vi "Detele_repeated.vi"(11 "timetags":u32[][](array[numeric])) -> (3 "detections":cluster{"time_ns":u32[], "q_photons":u32[]})   [LabVIEW 2014]
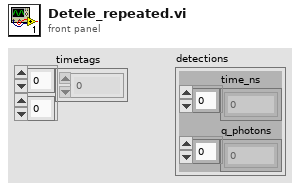
[diagram p1: front panel]
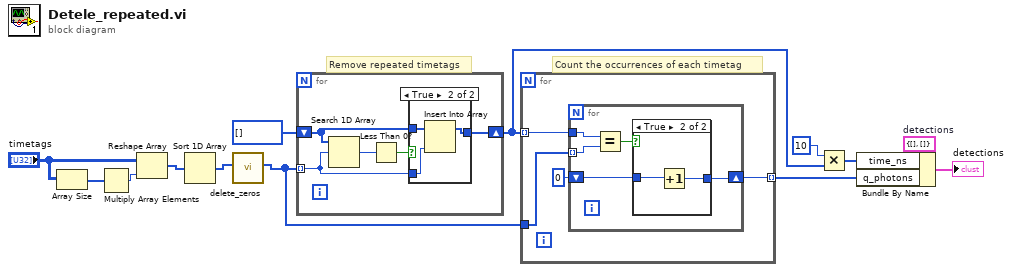
[diagram p0: block diagram]
diagram:
  w10 = cluster{"time_ns":u32[], "q_photons":u32[]} {"time_ns"=[], "q_photons"=[]}  # detections
  # "Count the occurrences of each timetag"
  # "Remove repeated timetags"
  n1 = Array Size(array="timetags") -> (size(s)=w7:i32[])
  n2 = Multiply Array Elements(1:w7) -> (0:w6:i32)
  n3 = Reshape Array("timetags", w6) -> (w13:u32[])
  n4 = Sort 1D Array(array=w13) -> (sorted array=w5:u32[])
  n5 = call "delete_zeros.vi"("array_in"=w5) -> ("array_out"=w4:u32[])  [unwired: 10 in]
  n6 = for {
    shift-right: [w14] -> w3
    shift-left: u32[] [] ("sorted array") -> [w16]
    tunnel: w4 -> [w15] mode=indexing
    n7 = Search 1D Array(1D array=w16, element=w15) -> (index of element=w18:i32)  [unwired: 1 in]
    n8 = Less Than 0?(x=w18) -> (x < 0?=w17:bool)
    n9 = case shown="True" w17 {
      tunnel: w16 -> [w19 w22]
      tunnel: w15 -> [_ w21]
      tunnel: [w19 w20] -> w14
      frame False {
      }
      frame True {
        n10 = Insert Into Array(array=w22, new element=w21) -> (w20:u32[])  [unwired: 1 in]
      }
    }
  }
  n11 = for {
    tunnel: w3 -> [w25] mode=indexing
    tunnel: w4 -> [w26]
    tunnel: [w23] -> w11 mode=indexing
    n12 = for {
      tunnel: w26 -> [w30] mode=indexing
      tunnel: w25 -> [w31]
      shift-right: [w27] -> w23
      shift-left: u32 0 ("Numeric") -> [w28]
      n13 = Equal?(x=w31, y=w30) -> (x = y?=w29:bool)
      n14 = case shown="True" w29 {
        tunnel: w28 -> [w32 w34]
        tunnel: [w32 w33] -> w27
        frame False {
        }
        frame True {
          n15 = Increment(x=w34) -> (x+1=w33:u32)
        }
      }
    }
  }
  n16 = Multiply(x=10, y=w3) -> (x*y=w2:u32[])
  n17 = Bundle By Name(cluster=w10, "time_ns"=w2, "q_photons"=w11) -> (→"detections":cluster{"time_ns":u32[], "q_photons":u32[]})
